vi "CLD 16 state machine solution.vi"() -> ()   [LabVIEW 2009]
doc: "CLD 16 exercise\n\nThis VI is mostly Event structure cases. The use of property nodes for enable and disable properties is a common occurence."
uses:
  CLD 16 Control Panel.ctl
  CLD 16 Status Panel.ctl
  CLD 16 state enum.ctl
  CLD 16 Data Cluster.ctl
panel:
  out "Line Two Active":bool
  out "Line One Active":bool
  out "Error Out":errorcluster
  in  "Error In":errorcluster
  in  "Stop Button":bool
  in  "Control Panel Line Two":T1 {"Tons of Peanuts" scale=0.0..10.0}
  out "Process Control":T2 {"Process Value" format="%#.3g"}
  in  "Control Panel Line One":T1 {"Tons of Peanuts" scale=0.0..10.0}
  # "Display Panel"
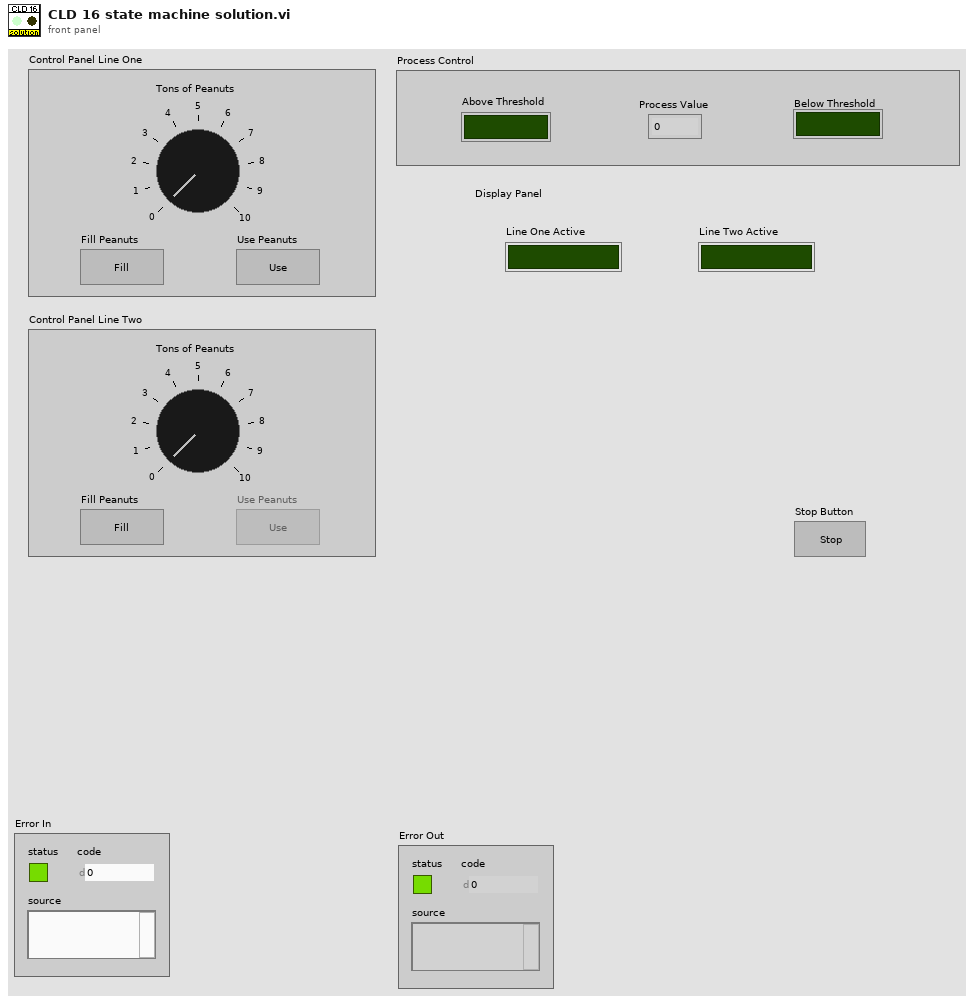
[diagram p1: front panel]
types:
  T1 = typedef "CLD 16 Control Panel.ctl" = cluster{"Tons of Peanuts":i8, "Fill Peanuts":bool, "Use Peanuts":bool}
  T2 = typedef "CLD 16 Status Panel.ctl" = cluster{"Above Threshold":bool, "Below Threshold":bool, "Process Value":dbl}
  T3 = typedef "CLD 16 Data Cluster.ctl" = cluster{"Control Panel Array":T1[], "Status Panel":T2, "Line One":bool, "Line Two":bool, "Stop Button":bool}
  T4 = typedef "CLD 16 state enum.ctl" = enum16{"initialize", "use", "idle"}
  T5 = enum8{"Enabled", "Disabled", "Disabled and Grayed Out"}
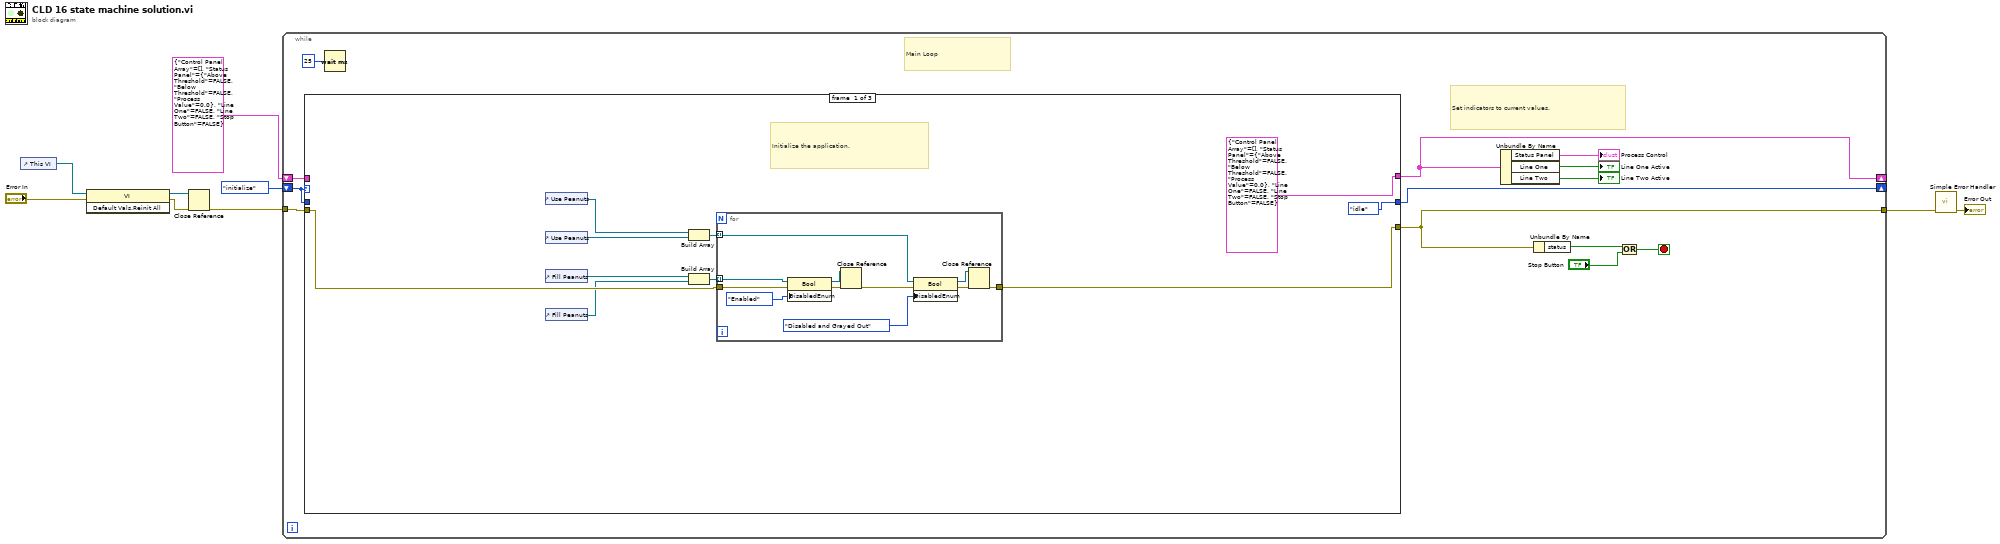
[diagram p0: block diagram]
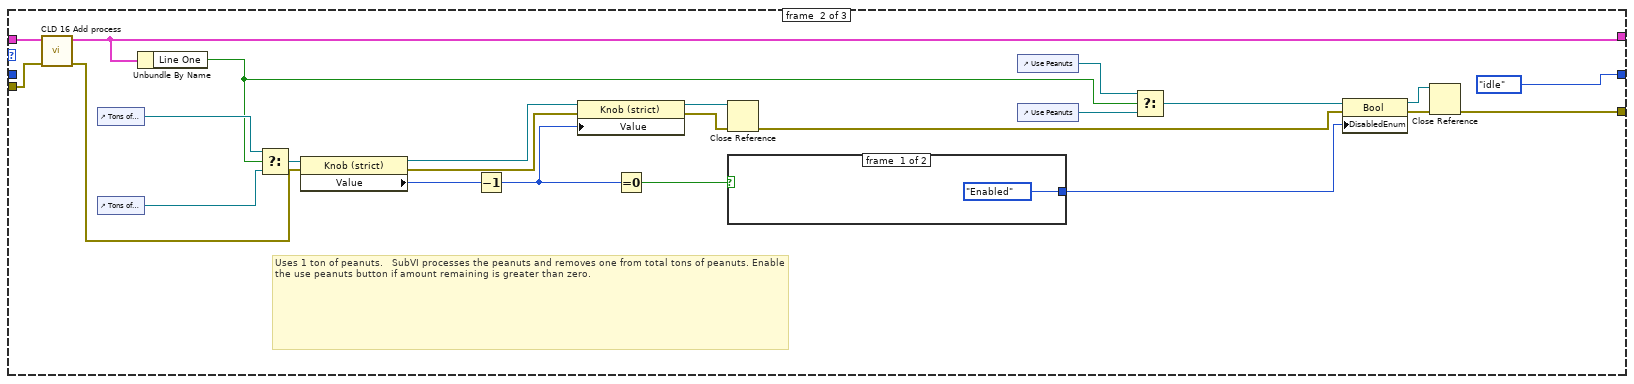
[diagram p2: hidden frame]
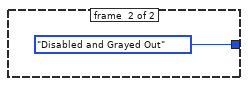
[diagram p3: hidden frame]
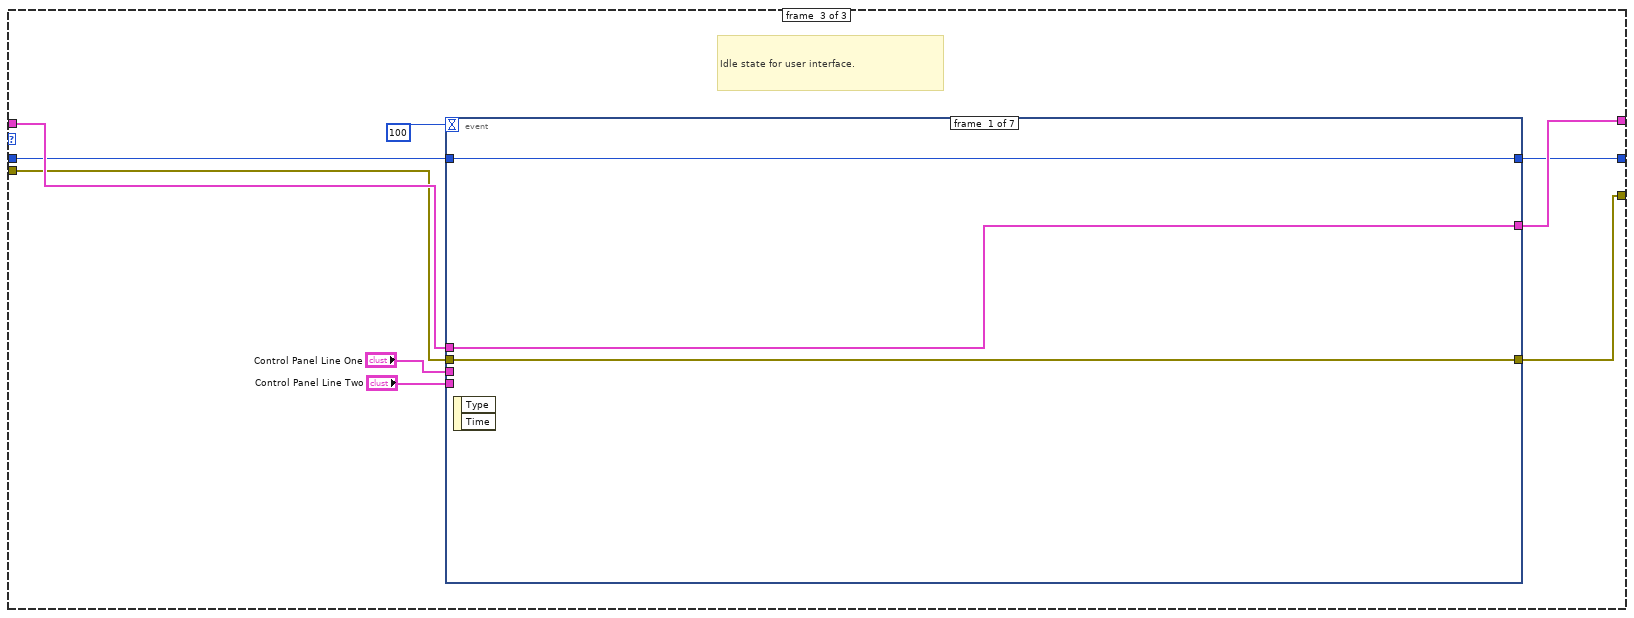
[diagram p4: hidden frame]
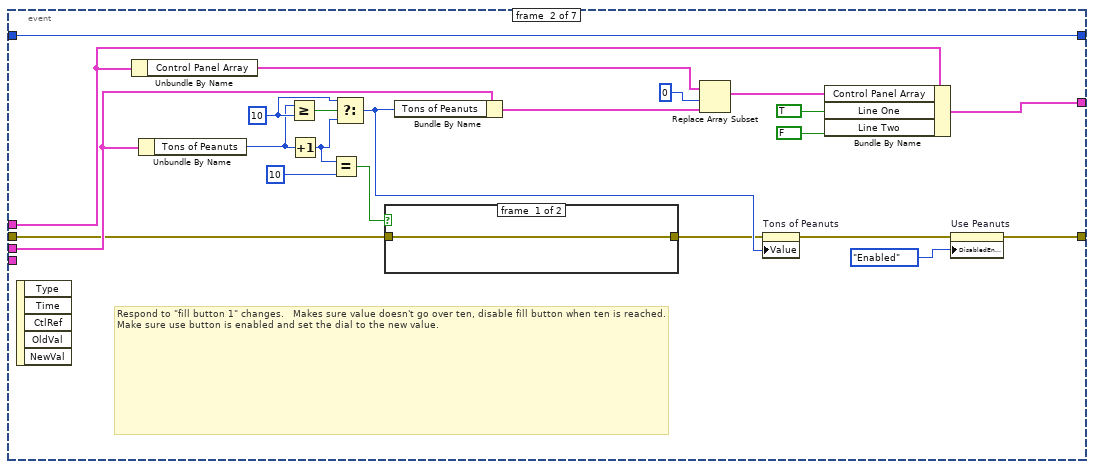
[diagram p5: hidden frame]
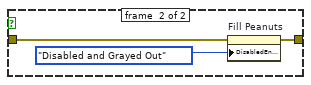
[diagram p6: hidden frame]
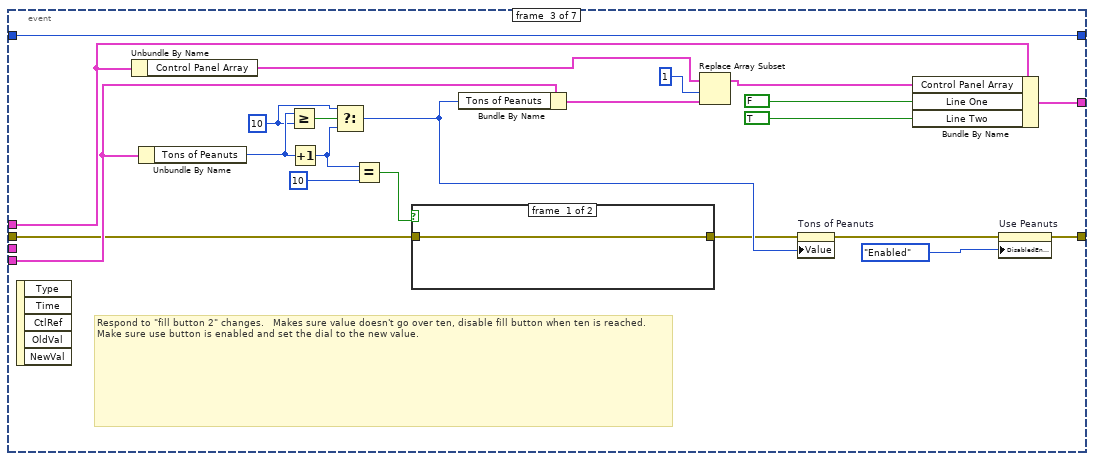
[diagram p7: hidden frame]
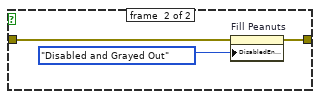
[diagram p8: hidden frame]
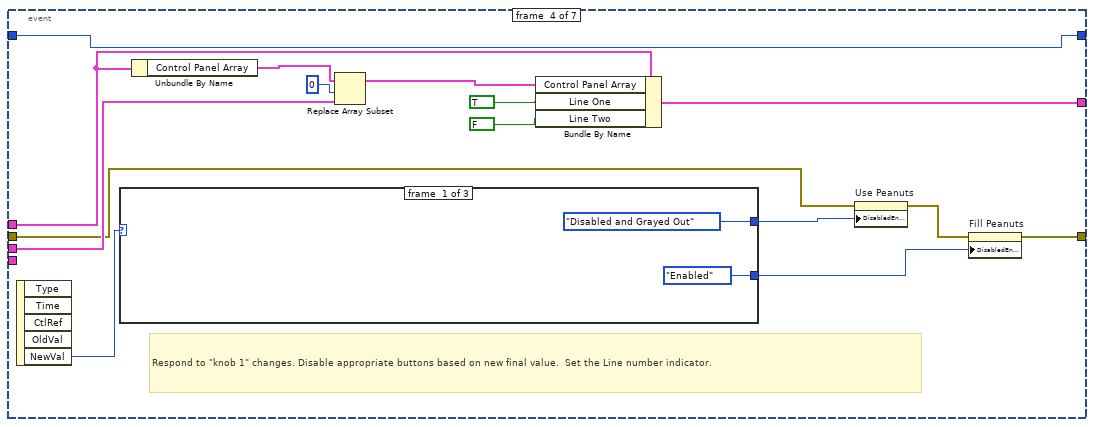
[diagram p9: hidden frame]
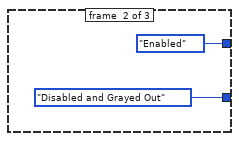
[diagram p10: hidden frame]
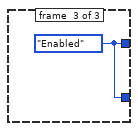
[diagram p11: hidden frame]
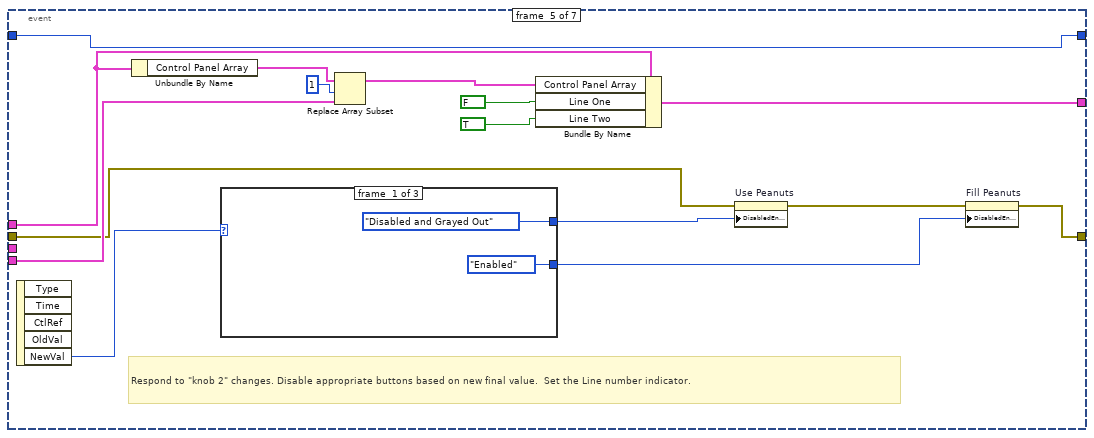
[diagram p12: hidden frame]
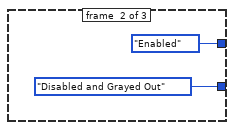
[diagram p13: hidden frame]
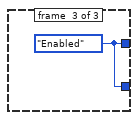
[diagram p14: hidden frame]
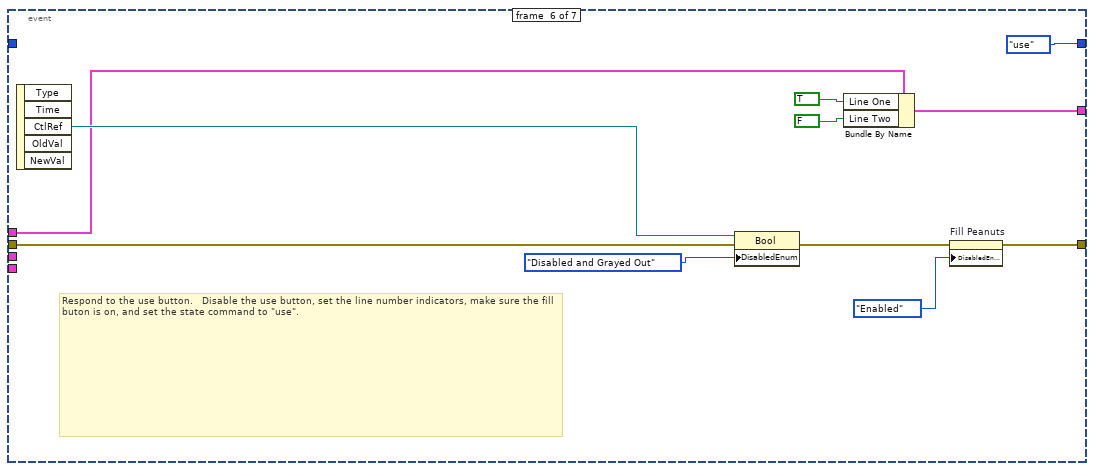
[diagram p15: hidden frame]
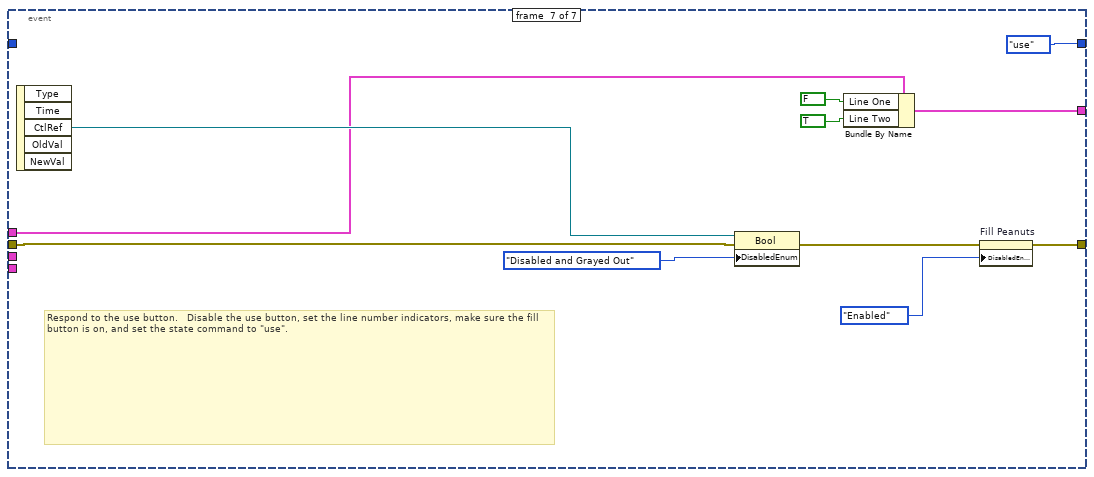
[diagram p16: hidden frame]
diagram:
  n1 = control-ref of="This VI"() -> (w4:refnum<vi>)
  n2 = invoke class="VI" method="Default Vals.Reinit All"(reference=w4, error in="Error In") -> (reference out=w2:refnum<vi>, error out=w5:errorcluster)  [unwired: 1 in, 1 out]
  n3 = Close Reference(reference=w2, error in (no error)=w5) -> (error out=w3:errorcluster)
  n4 = while {
    shift-right: [w21] -> _
    shift-left: CLD_16_state_enum."initialize" ("CLD 16 States") -> [w22]
    shift-right: [w14] -> _
    shift-left: T3 {"Control Panel Array"=[], "Status Panel"={"Above Threshold"=FALSE, "Below Threshold"=FALSE, "Process Value"=0.0}, "Line One"=FALSE, "Line Two"=FALSE, "Stop Button"=FALSE} ("Cluster") -> [w20]
    tunnel: [w18] -> w8
    tunnel: w3 -> [w19]
    stop <- w17 stop-if-true
    # "Main Loop"
    # "Set indicators to current values."
    n5 = case shown="\"use\"" w22 {
      tunnel: [CLD_16_state_enum."idle" ("CLD 16 States") CLD_16_state_enum."idle" ("CLD 16 States") w73] -> w21
      tunnel: w22 -> [_ _ w74]
      tunnel: w20 -> [_ w67 w78]
      tunnel: [T3 {"Control Panel Array"=[], "Status Panel"={"Above Threshold"=FALSE, "Below Threshold"=FALSE, "Process Value"=0.0}, "Line One"=FALSE, "Line Two"=FALSE, "Stop Button"=FALSE} ("Cluster") w65 w77] -> w14
      tunnel: [w27 w46 w70] -> w18
      tunnel: w19 -> [w28 w45 w71]
      frame #0 {
        # "Initialize the application."
        n6 = control-ref of="Use Peanuts"() -> (w30:refnum<vi>)
        n7 = control-ref of="Use Peanuts"() -> (w29:refnum<vi>)
        n8 = control-ref of="Fill Peanuts"() -> (w25:refnum<vi>)
        n9 = control-ref of="Fill Peanuts"() -> (w24:refnum<vi>)
        n10 = Build Array(w30, w29) -> (w31:refnum<vi>[])
        n11 = Build Array(w25, w24) -> (w23:refnum<vi>[])
        n12 = for {
          tunnel: w31 -> [w40] mode=indexing
          tunnel: w28 -> [w37]
          tunnel: [w39] -> w27
          tunnel: w23 -> [w38] mode=indexing
          n13 = property class="Bool"(reference=w38, error in=w37, "DisabledEnum"=T5."Enabled" ("Disabled")) -> (reference out=w33:refnum<vi>, error out=w36:errorcluster)
          n14 = Close Reference(reference=w33, error in (no error)=w36) -> (error out=w34:errorcluster)
          n15 = property class="Bool"(reference=w40, error in=w34, "DisabledEnum"=T5."Disabled and Grayed Out" ("Disabled")) -> (reference out=w42:refnum<vi>, error out=w43:errorcluster)
          n16 = Close Reference(reference=w42, error in (no error)=w43) -> (error out=w39:errorcluster)
        }
      }
      frame #1 {
        # "Uses 1 ton of peanuts.   SubVI processes the peanuts and removes one from total tons of peanuts. Enable the use peanuts button if amount remaining is greater than zero."
        n17 = call "CLD 16 Add process.vi"("error in (no error)"=w45, "Cluster in"=w67) -> ("error out"=w44:errorcluster, "Cluster out"=w65:T3)  [unwired: 8 in]
        n18 = control-ref of="Tons of Peanuts"() -> (w57:refnum<vi>)
        n19 = control-ref of="Tons of Peanuts"() -> (w58:refnum<vi>)
        n20 = Unbundle By Name(w65) -> ("Line One"=w56:bool)
        n21 = Select(t=w57, s=w56, f=w58) -> (s? t:f=w54:refnum<vi>)
        n22 = property class="Knob (strict)"(reference=w54, error in=w44) -> (reference out=w53:refnum<vi>, error out=w48:errorcluster, "Value"=w55:i8)
        n23 = Decrement(x=w55) -> (x-1=w50:i8)
        n24 = property class="Knob (strict)"(reference=w53, error in=w48, "Value"=w50) -> (reference out=w51:refnum<vi>, error out=w52:errorcluster)
        n25 = Equal To 0?(x=w50) -> (x = 0?=w49:bool)
        n26 = Close Reference(reference=w51, error in (no error)=w52) -> (error out=w47:errorcluster)
        n27 = case shown="True" w49 {
          tunnel: [T5."Enabled" ("Disabled") T5."Disabled and Grayed Out" ("Disabled")] -> w62
          frame #0 {
          }
          frame #1 {
          }
        }
        n28 = control-ref of="Use Peanuts"() -> (w64:refnum<vi>)
        n29 = control-ref of="Use Peanuts"() -> (w61:refnum<vi>)
        n30 = Select(t=w64, s=w56, f=w61) -> (s? t:f=w63:refnum<vi>)
        n31 = property class="Bool"(reference=w63, error in=w47, "DisabledEnum"=w62) -> (reference out=w59:refnum<vi>, error out=w60:errorcluster)
        n32 = Close Reference(reference=w59, error in (no error)=w60) -> (error out=w46:errorcluster)
      }
      frame #2 {
        # "Idle state for user interface."
        n33 = event shown="[1] \"Control Panel Line One.Fill Peanuts\": Value Change" {
          selector: _ -> [_ _ _ _ _ _ _]
          dyn-events: _ -> [_ _ _ _ _ _ _]
          timeout: 100 -> [_ _ _ _ _ _ _]
          tunnel: w78 -> [w80 w102 w128 w147 w167 w179 w190]
          tunnel: [w80 w103 w129 w148 w168 w178 w189] -> w77
          tunnel: "Control Panel Line One" -> [_ w95 _ w140 _ _ _]
          tunnel: [w81 w98 w124 w143 w163 CLD_16_state_enum."use" ("CLD 16 States") CLD_16_state_enum."use" ("CLD 16 States")] -> w73
          tunnel: w74 -> [w81 w98 w124 w143 w163 _ _]
          tunnel: "Control Panel Line Two" -> [_ _ w115 _ w158 _ _]
          tunnel: w71 -> [w79 w90 w114 w137 w157 w177 w188]
          tunnel: [w79 w88 w112 w135 w155 w175 w186] -> w70
          event #0 {
            n34 = event-data() -> ()  [unwired: 1 in, 2 out]
          }
          event #1 {
            w91 = i8 10 ("x")
            # "Respond to \"fill button 1\" changes.   Makes sure value doesn't go over ten, disable fill button when ten is reached. Make sure use button is enabled and set the dial to the new value."
            n35 = event-data() -> ()  [unwired: 1 in, 5 out]
            n36 = Unbundle By Name(w102) -> ("Control Panel Array"=w101:T1[])
            n37 = Unbundle By Name(w95) -> ("Tons of Peanuts"=w83:i8)
            n38 = Greater Or Equal?(x=w83, y=w91) -> (x >= y?=w86:bool)
            n39 = Increment(x=w83) -> (x+1=w82:i8)
            n40 = Equal?(x=w82, y=i8 10 ("x")) -> (x = y?=w84:bool)
            n41 = Select(t=w91, s=w86, f=w82) -> (s? t:f=w92:i8)
            n42 = case shown="True" w84 {
              tunnel: w90 -> [w104 w107]
              tunnel: [w104 w106] -> w87
              frame #0 {
              }
              frame #1 {
                n43 = property on="Fill Peanuts" class="Bool"(error in=w107, "DisabledEnum"=T5."Disabled and Grayed Out" ("Disabled")) -> (error out=w106:errorcluster)  [unwired: 1 in, 1 out]
              }
            }
            n44 = Bundle By Name(cluster=w95, "Tons of Peanuts"=w92) -> (w94:T1)
            n45 = Replace Array Subset(array=w101, new element=w94, index=0) -> (w99:T1[])
            n46 = property on="Tons of Peanuts" class="Knob (strict)"(error in=w87, "Value"=w92) -> (error out=w89:errorcluster)  [unwired: 1 in, 1 out]
            n47 = Bundle By Name(cluster=w102, "Control Panel Array"=w99, "Line One"=TRUE, "Line Two"=FALSE ("Line One")) -> (w103:T3)
            n48 = property on="Use Peanuts" class="Bool"(error in=w89, "DisabledEnum"=T5."Enabled" ("Disabled")) -> (error out=w88:errorcluster)  [unwired: 1 in, 1 out]
          }
          event #2 {
            w116 = i8 10 ("x")
            # "Respond to \"fill button 2\" changes.   Makes sure value doesn't go over ten, disable fill button when ten is reached. Make sure use button is enabled and set the dial to the new value."
            n49 = event-data() -> ()  [unwired: 1 in, 5 out]
            n50 = Unbundle By Name(w128) -> ("Control Panel Array"=w127:T1[])
            n51 = Unbundle By Name(w115) -> ("Tons of Peanuts"=w117:i8)
            n52 = Greater Or Equal?(x=w117, y=w116) -> (x >= y?=w119:bool)
            n53 = Increment(x=w117) -> (x+1=w110:i8)
            n54 = Select(t=w116, s=w119, f=w110) -> (s? t:f=w118:i8)
            n55 = Equal?(x=w110, y=i8 10 ("x")) -> (x = y?=w108:bool)
            n56 = case shown="True" w108 {
              tunnel: w114 -> [w130 w133]
              tunnel: [w130 w132] -> w109
              frame #0 {
              }
              frame #1 {
                n57 = property on="Fill Peanuts" class="Bool"(error in=w133, "DisabledEnum"=T5."Disabled and Grayed Out" ("Disabled")) -> (error out=w132:errorcluster)  [unwired: 1 in, 1 out]
              }
            }
            n58 = Bundle By Name(cluster=w115, "Tons of Peanuts"=w118) -> (w121:T1)
            n59 = Replace Array Subset(array=w127, new element=w121, index=1) -> (w125:T1[])
            n60 = property on="Tons of Peanuts" class="Knob (strict)"(error in=w109, "Value"=w118) -> (error out=w113:errorcluster)  [unwired: 1 in, 1 out]
            n61 = Bundle By Name(cluster=w128, "Control Panel Array"=w125, "Line One"=FALSE, "Line Two"=TRUE ("Line One")) -> (w129:T3)
            n62 = property on="Use Peanuts" class="Bool"(error in=w113, "DisabledEnum"=T5."Enabled" ("Disabled")) -> (error out=w112:errorcluster)  [unwired: 1 in, 1 out]
          }
          event #3 {
            # "Respond to \"knob 1\" changes. Disable appropriate buttons based on new final value.  Set the Line number indicator."
            n63 = event-data() -> ("NewVal"=w138:i8)  [unwired: 1 in, 4 out]
            n64 = case shown="10" w138 {
              tunnel: [T5."Disabled and Grayed Out" ("Disabled") T5."Enabled" ("Disabled") w153] -> w139
              tunnel: [T5."Enabled" ("Disabled") T5."Disabled and Grayed Out" ("Disabled") w153] -> w134
              frame #0 {
              }
              frame #1 {
              }
              frame #2 {
                w153 = T5."Enabled" ("Disabled")
              }
            }
            n65 = Unbundle By Name(w147) -> ("Control Panel Array"=w146:T1[])
            n66 = Replace Array Subset(array=w146, new element=w140, index=0) -> (w144:T1[])
            n67 = Bundle By Name(cluster=w147, "Control Panel Array"=w144, "Line One"=TRUE, "Line Two"=FALSE ("Line One")) -> (w148:T3)
            n68 = property on="Use Peanuts" class="Bool"(error in=w137, "DisabledEnum"=w139) -> (error out=w136:errorcluster)  [unwired: 1 in, 1 out]
            n69 = property on="Fill Peanuts" class="Bool"(error in=w136, "DisabledEnum"=w134) -> (error out=w135:errorcluster)  [unwired: 1 in, 1 out]
          }
          event #4 {
            # "Respond to \"knob 2\" changes. Disable appropriate buttons based on new final value.  Set the Line number indicator."
            n70 = event-data() -> ("NewVal"=w159:i8)  [unwired: 1 in, 4 out]
            n71 = Unbundle By Name(w167) -> ("Control Panel Array"=w166:T1[])
            n72 = case shown="1..9, Default" w159 {
              tunnel: [T5."Disabled and Grayed Out" ("Disabled") T5."Enabled" ("Disabled") w173] -> w160
              tunnel: [T5."Enabled" ("Disabled") T5."Disabled and Grayed Out" ("Disabled") w173] -> w154
              frame #0 {
              }
              frame #1 {
              }
              frame #2 {
                w173 = T5."Enabled" ("Disabled")
              }
            }
            n73 = Replace Array Subset(array=w166, new element=w158, index=1) -> (w164:T1[])
            n74 = Bundle By Name(cluster=w167, "Control Panel Array"=w164, "Line One"=FALSE, "Line Two"=TRUE ("Line One")) -> (w168:T3)
            n75 = property on="Use Peanuts" class="Bool"(error in=w157, "DisabledEnum"=w160) -> (error out=w156:errorcluster)  [unwired: 1 in, 1 out]
            n76 = property on="Fill Peanuts" class="Bool"(error in=w156, "DisabledEnum"=w154) -> (error out=w155:errorcluster)  [unwired: 1 in, 1 out]
          }
          event #5 {
            # "Respond to the use button.   Disable the use button, set the line number indicators, make sure the fill buton is on, and set the state command to \"use\"."
            n77 = event-data() -> ("CtlRef"=w183:refnum<vi>)  [unwired: 1 in, 4 out]
            n78 = property class="Bool"(reference=w183, error in=w177, "DisabledEnum"=T5."Disabled and Grayed Out" ("Disabled")) -> (error out=w176:errorcluster)  [unwired: 1 out]
            n79 = Bundle By Name(cluster=w179, "Line One"=TRUE, "Line Two"=FALSE ("Line One")) -> (w178:T3)
            n80 = property on="Fill Peanuts" class="Bool"(error in=w176, "DisabledEnum"=T5."Enabled" ("Disabled")) -> (error out=w175:errorcluster)  [unwired: 1 in, 1 out]
          }
          event #6 {
            # "Respond to the use button.   Disable the use button, set the line number indicators, make sure the fill button is on, and set the state command to \"use\"."
            n81 = event-data() -> ("CtlRef"=w194:refnum<vi>)  [unwired: 1 in, 4 out]
            n82 = property class="Bool"(reference=w194, error in=w188, "DisabledEnum"=T5."Disabled and Grayed Out" ("Disabled")) -> (error out=w187:errorcluster)  [unwired: 1 out]
            n83 = Bundle By Name(cluster=w190, "Line One"=FALSE, "Line Two"=TRUE ("Line One")) -> (w189:T3)
            n84 = property on="Fill Peanuts" class="Bool"(error in=w187, "DisabledEnum"=T5."Enabled" ("Disabled")) -> (error out=w186:errorcluster)  [unwired: 1 in, 1 out]
          }
        }
      }
    }
    n85 = Wait (ms)(milliseconds to wait=u32 25) -> ()  [unwired: 1 out]
    n86 = Unbundle By Name(w14) -> ("Status Panel"=→"Process Control":T2, "Line One"=→"Line One Active":bool, "Line Two"=→"Line Two Active":bool)
    n87 = Unbundle By Name(w18) -> ("status"=w15:bool)
    n88 = Or(x=w15, y="Stop Button") -> (x .or. y?=w17:bool)
  }
  n89 = call <vilib>:"Simple Error Handler.vi"("error in (no error)"=w8) -> ("error out"=→"Error Out":errorcluster)  [unwired: 4 in, 4 out]
